vi "Chirp_subVI.vi"(6 "# Output Samples":i16, 9 "Initial Frequency (Hz)":dbl, 10 "Final Frequency (Hz)":dbl, 11 "Amplitude (V)":dbl) -> (3 "Chirp":fxp<+,16,3>[](array[numeric]))   [LabVIEW 2017]
doc: "Outputs a linear, frequency modulated chirp."
uses:
  <vilib>/Analysis/4window.llb/Hanning Window (DBL).vi
  <vilib>/Analysis/4window.llb/AllCosWindow (DBL).vi
  <vilib>/Analysis/NI_AALPro.lvlib
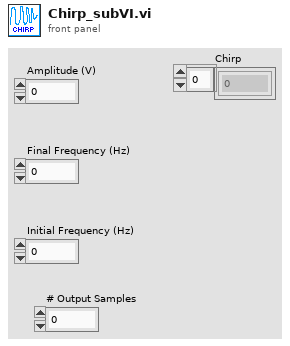
[diagram p1: front panel]
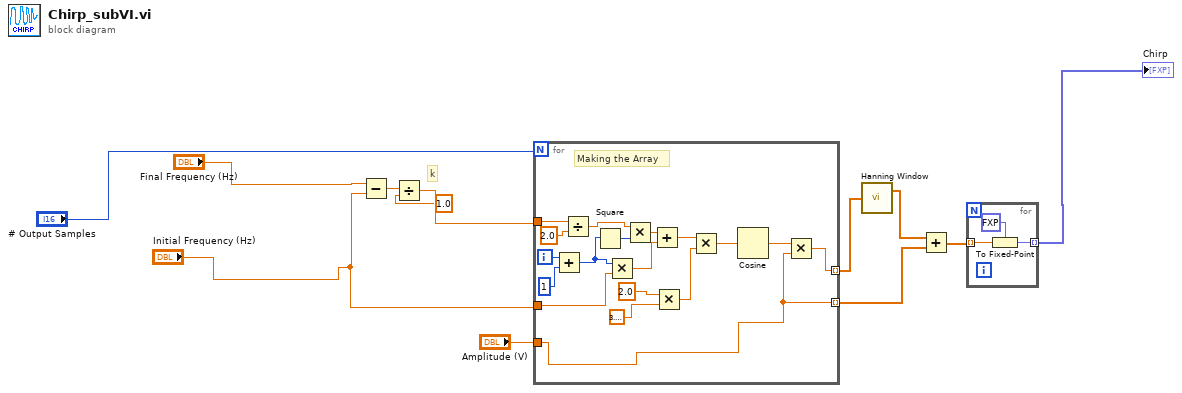
[diagram p0: block diagram]
diagram:
  # "k"
  n1 = Subtract(x="Final Frequency (Hz)", y="Initial Frequency (Hz)") -> (x-y=w5:dbl)
  n2 = Divide(x=w5, y=1.0) -> (x/y=w8:dbl)
  n3 = for {
    N: "# Output Samples" -> [_]
    tunnel: w8 -> [w30]
    tunnel: [w15] -> w6 mode=indexing
    tunnel: "Initial Frequency (Hz)" -> [w16]
    tunnel: [w13] -> w11 mode=indexing
    tunnel: "Amplitude (V)" -> [w13]
    i -> [w27]
    # "Making the Array"
    n4 = Add(x=w27, y=1) -> (x+y=w14:i32)
    n5 = Divide(x=w30, y=2.0) -> (x/y=w17:dbl)
    n6 = Square(x=w14) -> (x^2=w18:i32)
    n7 = Multiply(x=w14, y=w16) -> (x*y=w24:dbl)
    n8 = Multiply(x=w17, y=w18) -> (x*y=w28:dbl)
    n9 = Add(x=w28, y=w24) -> (x+y=w23:dbl)
    n10 = Multiply(x=sgl 2.0, y=sgl 3.1415927) -> (x*y=w20:dbl)
    n11 = Multiply(x=w23, y=w20) -> (x*y=w19:dbl)
    n12 = Cosine(x=w19) -> (cos(x)=w25:dbl)
    n13 = Multiply(x=w25, y=w13) -> (x*y=w15:dbl)
  }
  n14 = call-poly <vilib>:"Hanning Window.vi"("X"=w6) -> ("Windowed X"=w10:dbl[])  [unwired: 1 out]
  n15 = Add(x=w10, y=w11) -> (x+y=w12:dbl[])
  n16 = for {
    tunnel: w12 -> [w32] mode=indexing
    tunnel: [w31] -> w4 mode=indexing
    n17 = To Fixed-Point(fixed-point type=fxp<+,16,3> 0.0 ("AO0"), number=w32) -> (fixed-point=w31:fxp<+,16,3>)
  }
  "Chirp" <- w4
